vi "Dequeue Command.vi"(7 "Wait? (T)":bool=TRUE, 8 "error in (no error)":errorcluster, 11 "Websocket Client in":refnum<class "Websocket Client.lvclass">) -> (0 "error out":errorcluster, 1 "timed out?":bool, 2 "Command":T1, 3 "Websocket Client out":refnum<class "Websocket Client.lvclass">)   [LabVIEW 2020, in "Stream-Websocket.lvlib" / "Websocket Client.lvclass"]
uses:
  Websocket Client.lvclass
  Websocket Client.lvclass/Websocket Client.ctl
  Client Command.ctl
  Stream-Websocket.lvlib
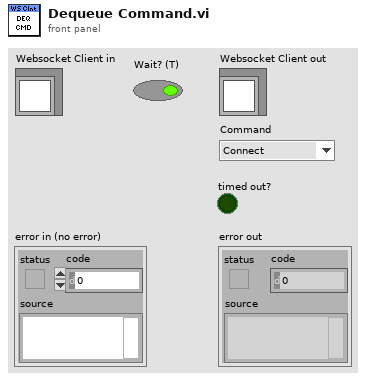
[diagram p1: front panel]
types:
  T1 = typedef "Stream-Websocket.lvlib/Client Command.ctl" = enum16{"Connect", "Close", "Shutdown", "Reconnect"}
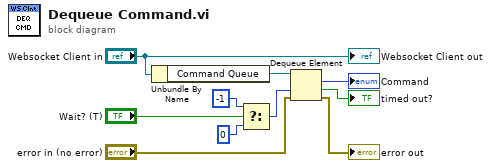
[diagram p0: block diagram]
diagram:
  n1 = Unbundle By Name("Websocket Client in") -> ("Command Queue"=w9:refnum<queue>)
  n2 = Select(t=-1, s="Wait? (T)", f=0) -> (s? t:f=w1:i32)
  n3 = Dequeue Element(queue=w9, timeout in ms (-1)=w1, error in (no error)="error in (no error)") -> (element=→"Command":T1, timed out?=→"timed out?":bool, error out=→"error out":errorcluster)  [unwired: 1 out]
  "Websocket Client out" <- "Websocket Client in"
